vi "example_GCommand.vi"() -> ()   [LabVIEW 2020]
uses:
  resources/gclib32/gclib32.lvlib
panel:
  out "Error Out":errorcluster
  in  "IP Address":string="192.168.1.77"
  out "Response":string="\r\n:"
  in  "Command":string="MG TIME"
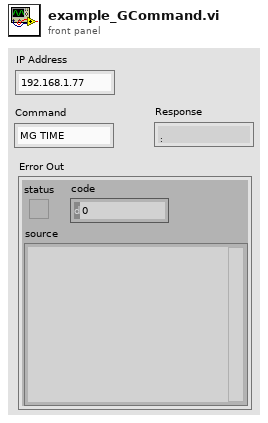
[diagram p1: front panel]
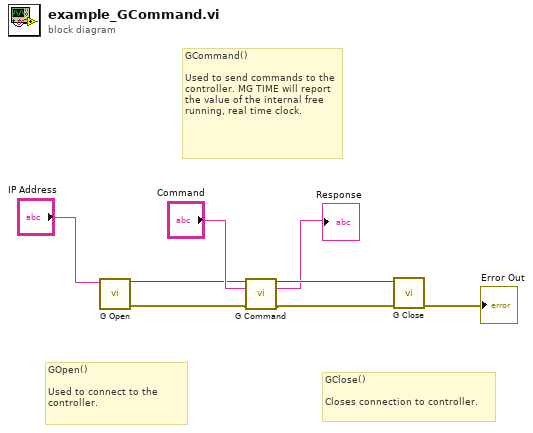
[diagram p0: block diagram]
diagram:
  # "GClose()\n\nCloses connection to controller."
  # "GCommand()\n\nUsed to send commands to the controller. MG TIME will report the value of the internal free running, real time clock."
  # "GOpen()\n\nUsed to connect to the controller."
  n1 = call "G Open.vi"("address"="IP Address") -> ("error out"=w2:errorcluster, "g out"=w3:u32)  [unwired: 8 in]
  n2 = call "G Command.vi"("g"=w3, "command"="Command", "error in (no error)"=w2) -> ("g out"=w7:u32, "buffer out"=→"Response":string, "error out"=w4:errorcluster)  [unwired: 10 in]
  n3 = call "G Close.vi"("error in (no error)"=w4, "g"=w7) -> ("error out"=→"Error Out":errorcluster)  [unwired: 9 in]
